vi "Performance Test.vi"() -> ()   [LabVIEW 2021]
uses:
  CIFChannels/Typedef/Direction.ctl
  CIF_NIChn_Fifo_Power_DVR.lvclass
  D:/dev/CIF-LVCore/src/Channels/CIFChannels/CIFChannels.lvclass
  D:/dev/CIF-LVCore/src/Channels/CIF_NIChn/NIChn/CIF_NIChn.lvclass
  ChannelCommon/typedef/FIFO Config.ctl
  <vilib>/Platform/TimedLoop/XDataNode/timing_clust.ctl
  <vilib>/Platform/TimedLoop/XDataNode/nitl_modes.ctl
  <vilib>/Platform/TimedLoop/XDataNode/wakeup.ctl
  ChannelCommon/typedef/TimeStamps.ctl
  ChannelCommon/typedef/Datatype Power Waveform.ctl
  CIF_NIChn_Fifo_Power_DVR.lvclass/CIF_NIChn_Fifo_Power_DVR.ctl
  ChannelCommon/CIFFIFO/CIFfifo.lvclass/CIFfifo.ctl
  NIChn/CIF_NIChn.lvclass/CIF_NIChn.ctl
  CIFChannels/CIFChannels.lvclass/CIFChannels.ctl
  CIFCore/Common/Utilities/Add Error.vi
  SubVIs/Get DVR From Circular Buffer.vi
  Core/Write Power DVR FIFO Direct Dispatch.vi
  Core/Read Power DVR FIFO Direct Dispatch.vi
  CIFCore/Common/Utilities/Append Error Location.vi
  ChannelCommon/Utilities/Get Waveform DVRs.vi
  <vilib>/CIFChannels/Top Level/Write Variable Length U8 Array.vi
  NIChn/Accessors/Read CIF Channel.vi
  NIChn/Accessors/Write CIF Channel.vi
  SubVIs/Flatten.vi
  ChannelCommon/CIFFIFO/Accessors/Read Length.vi
  NIChn/SubVIs/Check Disconnect.vi
  <vilib>/CIFChannels/Top Level/Read Variable Length U8 Array.vi
  SubVIs/Unflatten.vi
  CIFChannels/Accessors/Read Channel State.vi
  CIFChannels/Accessors/Read Direction.vi
  <vilib>/CIFChannels/SubVIs/Get dll Path.vi
  ChannelCommon/CIFFIFO/Utilities/Update Header.vi
  ChannelCommon/CIFFIFO/Flatten/DVR Flatten.vi
  ChannelCommon/CIFFIFO/Accessors/Write T0.vi
  ChannelCommon/CIFFIFO/Accessors/Write T_Out.vi
  ChannelCommon/CIFFIFO/Accessors/Write ClockID.vi
  CIFChannels/Accessors/Write Channel State.vi
  CIFChannels/Accessors/Read Disconnect Behavior.vi
  <vilib>/CIFChannels/Top Level/Read Variable Length U8 Array.vi/81056090-23cf-424a-a716-29db01c8ef1b.vi
  <vilib>/CIFChannels/Top Level/Read Variable Length U8 Array.vi/6610cd62-0a6d-4591-8fd4-6453482a4bc1.vi
  <vilib>/CIFChannels/Top Level/Read Variable Length U8 Array.vi/93d598b0-524b-4f76-9570-a74a86ef2c6f.vi
  ChannelCommon/CIFFIFO/Accessors/Write Timeout.vi
  ChannelCommon/CIFFIFO/Flatten/DVR Unflatten.vi
  ChannelCommon/CIFFIFO/Accessors/Read Header.vi
  ChannelCommon/CIFFIFO/Accessors/Write Header.vi
  ChannelCommon/Utilities/Flatten Header.vi
  ChannelCommon/CIFFIFO/Flatten/DVR Flatten.vi/6fdbece9-bad6-4a8e-9bf7-fe1528478dd6.vi
  ChannelCommon/CIFFIFO/Accessors/Write Payload Length.vi
  <vilib>/CIFChannels/Top Level/Read Variable Length U8 Array.vi/81056090-23cf-424a-a716-29db01c8ef1b.vi/4bc1c15b-36ab-481f-b8dd-c64075ce723a.vi
  <vilib>/CIFChannels/Top Level/Read Variable Length U8 Array.vi/81056090-23cf-424a-a716-29db01c8ef1b.vi/d83cb72b-7713-41fc-a3d1-682de79cf574.vi
  <vilib>/CIFChannels/Top Level/Read Variable Length U8 Array.vi/6610cd62-0a6d-4591-8fd4-6453482a4bc1.vi/c28b0ead-42ad-4072-80a2-aca7f2bd7ce3.vi
  <vilib>/CIFChannels/Top Level/Read Variable Length U8 Array.vi/93d598b0-524b-4f76-9570-a74a86ef2c6f.vi/4bc1c15b-36ab-481f-b8dd-c64075ce723a.vi
  <vilib>/CIFChannels/Top Level/Read Variable Length U8 Array.vi/93d598b0-524b-4f76-9570-a74a86ef2c6f.vi/d83cb72b-7713-41fc-a3d1-682de79cf574.vi
  ChannelCommon/Utilities/Unflatten Header.vi
  ChannelCommon/CIFFIFO/Flatten/DVR Flatten.vi/6fdbece9-bad6-4a8e-9bf7-fe1528478dd6.vi/c28b0ead-42ad-4072-80a2-aca7f2bd7ce3.vi
  NIChn/CIF_NIChn.lvclass
  ChannelCommon/Utilities/Update Time.vi
  <vilib>/Platform/TimedLoop/XDataNode/XDataNode.xnode
  <vilib>/Platform/TimedLoop/XDataNode/XDNodeRunTimeDep.lvlib
  CIFChannels/CIFChannels.lvclass
  ChannelCommon/ChannelCommon.lvlib
panel:
  out "avg TO":dbl
  out "max TO":dbl
  out "timed out? 3":bool
  out "timed out?":bool
  out "avg channel":dbl
  out "max channel":dbl
  out "pass":bool
  out "error out":errorcluster
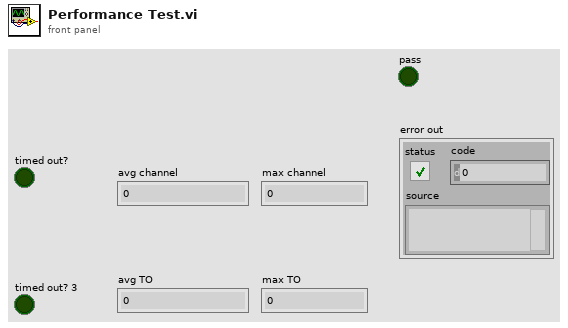
[diagram p1: front panel]
types:
  T1 = typedef "ChannelCommon.lvlib/FIFO Config.ctl" = cluster{"Depth":u64, "Flags":u64, "ClockID":u8}
  T2 = typedef "CIFChannels.lvclass/Direction.ctl" = enum16{"Publisher", "Subscriber"}
  T3 = typedef "ChannelCommon.lvlib/Datatype Power Waveform.ctl" = cluster{"Voltage":dbl[], "Current":dbl[], "dT":dbl, "Timestamp":u64, "Read Lock":bool}
  T4 = typedef "ChannelCommon.lvlib/TimeStamps.ctl" = cluster{"ClockID":u8, "T0":u64, "T_Out":u64}
  T5 = typedef "XDNodeRunTimeDep.lvlib/timing_clust.ctl" = cluster{"Expected End [f-1]":u64, "Actual End [f-1]":u64, "Finished Late? [f-1]":bool, "Expected End [i-1]":u64, "Actual End [i-1]":u64, "Finished Late? [i-1]":bool, "Expected Start [i]":u64, "Actual Start [i]":u64, "Expected Start [f]":u64, "Actual Start [f]":u64, "Source Name":string, "Structure Name":string, "Period":i64, "Deadline":i64, "Offset":i64, "Start":i64, "Priority":i32, "Timeout":i32, "Mode":T6, "Wakeup Reason":T7, "Error":errorcluster, "Source Type":string, "Secondary Source Type":string, "Global End Time":u64, "Global Start Time":u64, "Frame Duration":u64, "Iteration Duration":u64, "Assigned CPU":i32, "I/O Scan Engine Mode":u32}
  T6 = typedef "XDNodeRunTimeDep.lvlib/nitl_modes.ctl" = enum32{"No Change", "Process missed periods, maintain original phase", "Discard missed periods, maintain original phase", "Process missed periods, ignore original phase", "Discard missed periods, ignore original phase"}
  T7 = typedef "XDNodeRunTimeDep.lvlib/wakeup.ctl" = enum32{"Normal", "Aborted", "Asynchronous wakeup", "Timing source error", "Timed loop error", "Timeout"}
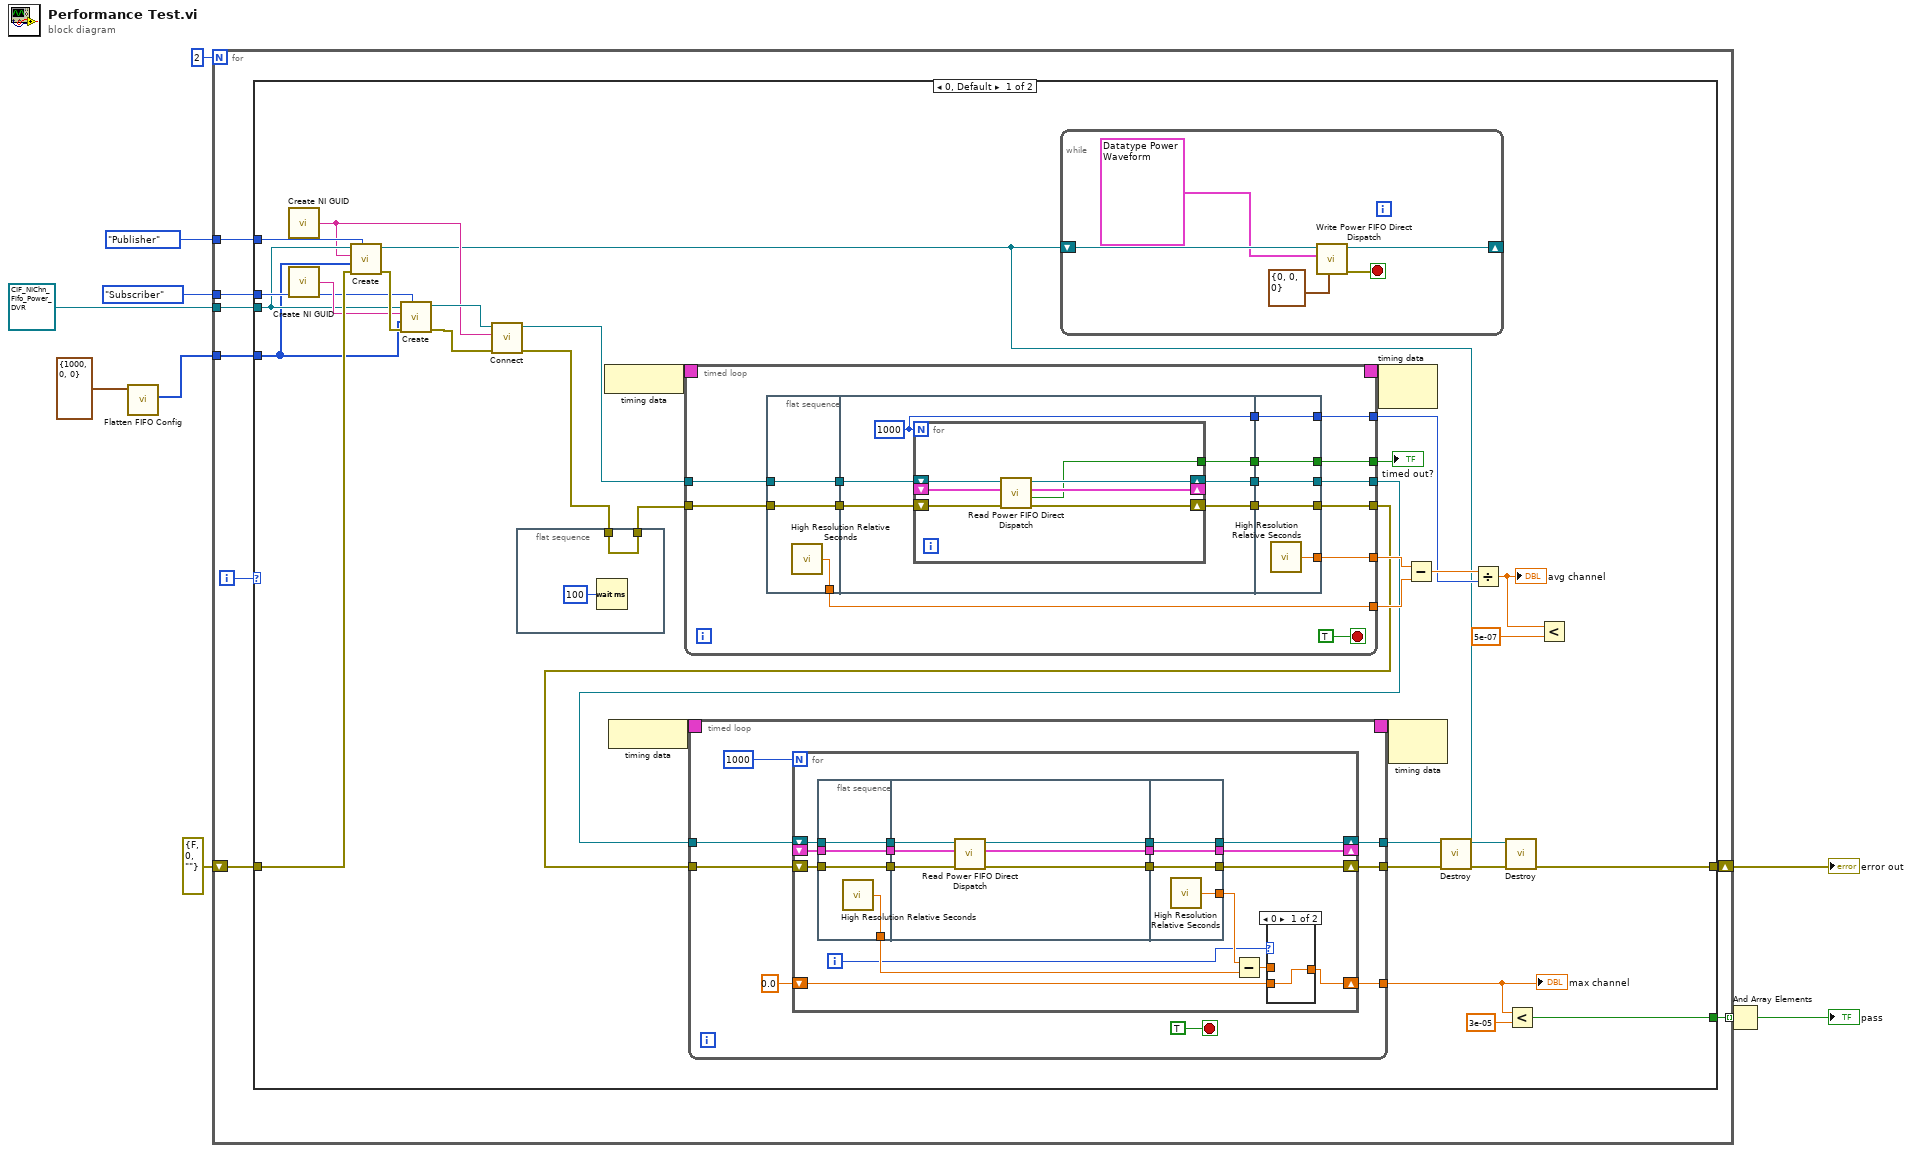
[diagram p0: block diagram]
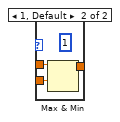
[diagram p2: hidden frame]
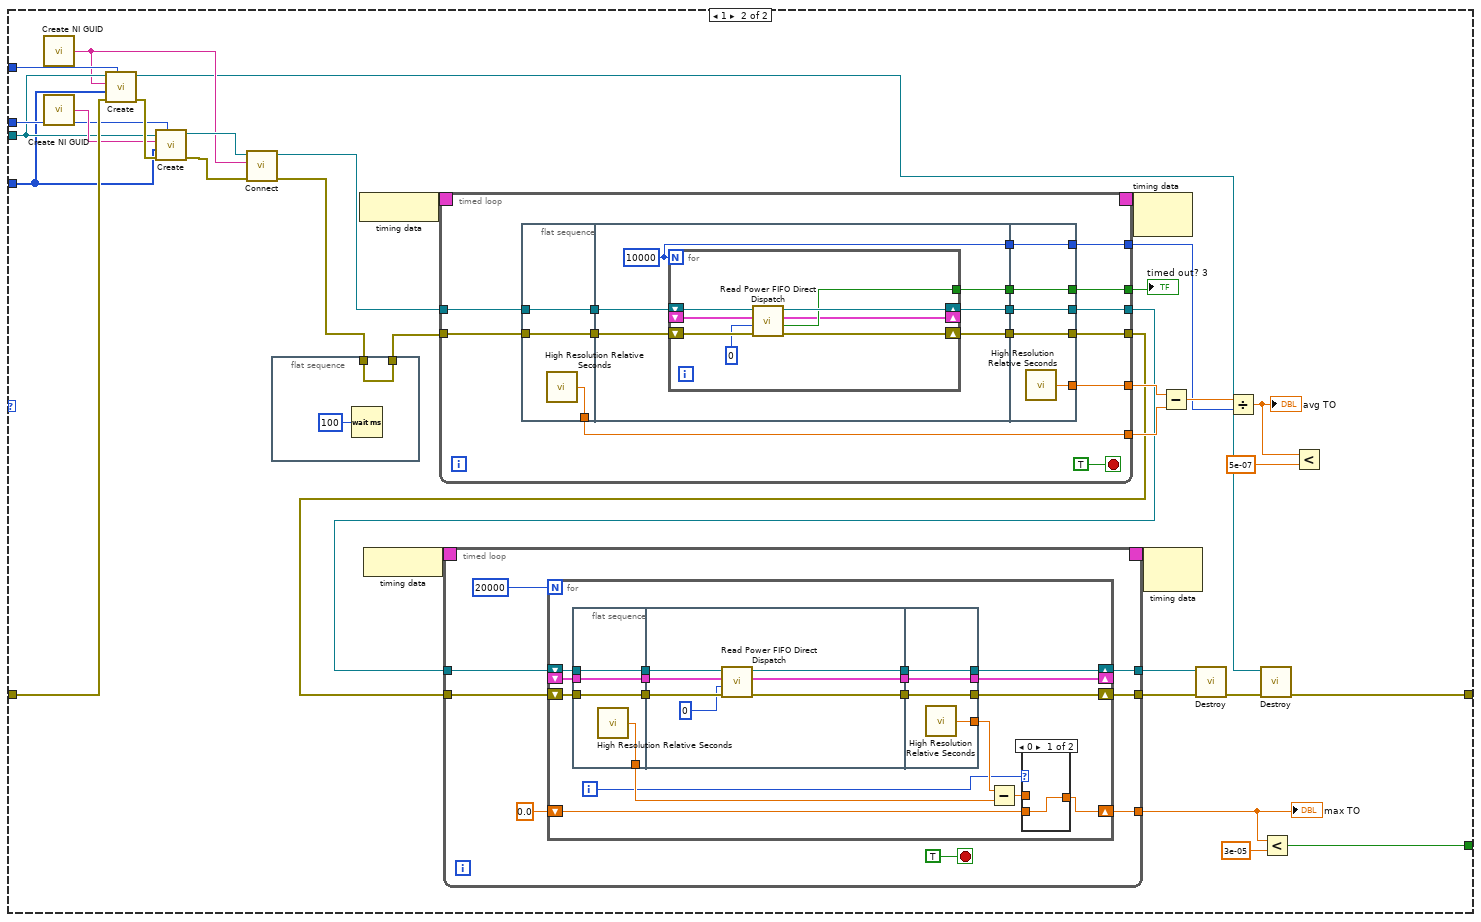
[diagram p3: hidden frame]
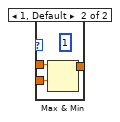
[diagram p4: hidden frame]
diagram:
  n1 = call "Flatten FIFO Config.vi"("FIFO Config in"=T1 {"Depth"=1000, "Flags"=0, "ClockID"=0}) -> ("Flattened Data out"=w2:u8[])  [unwired: 8 in, 2 out]
  n2 = for {
    N: 2 -> [_]
    tunnel: [w18] -> w8 mode=indexing
    shift-right: [w17] -> w10
    shift-left: errorcluster {"status"=FALSE, "code"=0, "source"=""} ("error out") -> [w15]
    tunnel: Direction."Publisher" ("Direction") -> [w14]
    tunnel: Direction."Subscriber" ("Direction") -> [w13]
    tunnel: refnum<class "CIF_NIChn_Fifo_Power_DVR.lvclass"> refnum ("CIF_NIChn_Fifo_Power.lvclass") -> [w12]
    tunnel: w2 -> [w11]
    i -> [w16]
    n3 = case shown="0, Default" w16 {
      tunnel: [w38 w167] -> w18
      tunnel: [w22 w151] -> w17
      tunnel: w15 -> [w36 w165]
      tunnel: w14 -> [w34 w163]
      tunnel: w13 -> [w33 w162]
      tunnel: w12 -> [w32 w161]
      tunnel: w11 -> [w28 w157]
      frame 0, Default {
        n4 = call <vilib>:"Create NI GUID.vi"() -> ("NI GUID"=w30:string)
        n5 = call <vilib>:"Create NI GUID.vi"() -> ("NI GUID"=w35:string)
        n6 = call-dynamic "Create.vi"("Direction"=w34, "error in (no error)"=w36, "Custom Config Data"=w28, "Name"=w30, "CIFTag in"=w32) -> ("error out"=w37:errorcluster, "CIFTag out"=w23:refnum<class "CIF_NIChn_Fifo_Power_DVR.lvclass">)  [unwired: 5 in]
        n7 = call-dynamic "Create.vi"("Direction"=w33, "error in (no error)"=w37, "Custom Config Data"=w28, "Name"=w35, "CIFTag in"=w32) -> ("error out"=w29:errorcluster, "CIFTag out"=w31:refnum<class "CIF_NIChn_Fifo_Power_DVR.lvclass">)  [unwired: 5 in]
        n8 = call-dynamic "Connect.vi"("error in (no error)"=w29, "Connection Name"=w30, "CIFTag in"=w31) -> ("error out"=w21:errorcluster, "CIFTag out"=w27:refnum<class "CIF_NIChn_Fifo_Power_DVR.lvclass">)  [unwired: 7 in]
        n9 = flat-sequence {
          tunnel: w21 -> [w54]
          tunnel: [w54] -> w20
          frame #0 {
            n10 = Wait (ms)(milliseconds to wait=u32 100) -> ()  [unwired: 1 out]
          }
        }
        n11 = node-c288() -> (w52:T5)
        n12 = node-c288() -> (w50:T5)
        n13 = timed-loop {
          timing: w52 -> [_]
          timing-out: [_] -> w51
          tunnel: w27 -> [w122]
          tunnel: w20 -> [w121]
          tunnel: [w117] -> w44
          tunnel: [w115] -> w43
          tunnel: [w113] -> w48
          tunnel: [w112] -> w47
          tunnel: [w111] -> w45
          tunnel: [w109] -> w19
          stop <- TRUE stop-if-true
          n14 = flat-sequence {
            tunnel: w121 -> [w124]
            tunnel: w122 -> [w125]
            tunnel: [w125] -> w119
            tunnel: [w124] -> w118
            tunnel: [w123] -> w112
            tunnel: w119 -> [w131]
            tunnel: w118 -> [w130]
            tunnel: [w129] -> w116
            tunnel: [w128] -> w114
            tunnel: [w127] -> w110
            tunnel: [w126] -> w108
            tunnel: [w143] -> w117
            tunnel: w116 -> [w143]
            tunnel: [w142] -> w115
            tunnel: w114 -> [w142]
            tunnel: [w141] -> w113
            tunnel: [w140] -> w111
            tunnel: w110 -> [w140]
            tunnel: [w139] -> w109
            tunnel: w108 -> [w139]
            frame #0 {
              n15 = call <vilib>:"High Resolution Relative Seconds.vi"() -> ("relative seconds"=w123:dbl)
            }
            frame #1 {
              w127 = 1000
              n16 = for {
                N: w127 -> [_]
                shift-right: [w133] -> w129
                shift-left: w131 -> [w138]
                shift-right: [w136] -> w128
                shift-left: w130 -> [w137]
                shift-right: [w135] -> _
                shift-left: _ -> [w134]
                tunnel: [w132] -> w126
                n17 = call "Read Power FIFO Direct Dispatch.vi"("error in (no error)"=w137, "Power Waveform In"=w134, "CIFTag in"=w138) -> ("error out"=w136:errorcluster, "timed out?"=w132:bool, "Power Waveform Out"=w135:T3, "CIFTag out"=w133:refnum<class "CIF_NIChn_Fifo_Power_DVR.lvclass">)  [unwired: 4 in, 1 out]
              }
            }
            frame #2 {
              n18 = call <vilib>:"High Resolution Relative Seconds.vi"() -> ("relative seconds"=w141:dbl)
            }
          }
        }
        "timed out?" <- w19
        n19 = timed-loop {
          timing: w50 -> [_]
          timing-out: [_] -> w49
          tunnel: w44 -> [w67]
          tunnel: w43 -> [w66]
          tunnel: [w64] -> w26
          tunnel: [w63] -> w25
          tunnel: [w60] -> w40
          stop <- TRUE stop-if-true
          n20 = for {
            N: 1000 -> [_]
            shift-right: [w79] -> w64
            shift-left: w67 -> [w81]
            shift-right: [w78] -> w63
            shift-left: w66 -> [w80]
            shift-right: [w72] -> w60
            shift-left: 0.0 -> [w73]
            shift-right: [w71] -> _
            shift-left: _ -> [w77]
            i -> [w69]
            n21 = flat-sequence {
              tunnel: w80 -> [w92]
              tunnel: w81 -> [w93]
              tunnel: [w93] -> w85
              tunnel: [w92] -> w84
              tunnel: [w91] -> w75
              tunnel: w77 -> [w90]
              tunnel: [w90] -> w83
              tunnel: w85 -> [w99]
              tunnel: w84 -> [w98]
              tunnel: [w95] -> w82
              tunnel: w83 -> [w94]
              tunnel: [w96] -> w70
              tunnel: [w97] -> w68
              tunnel: [w103] -> w79
              tunnel: w82 -> [w103]
              tunnel: [w102] -> w78
              tunnel: [w101] -> w76
              tunnel: [w100] -> w71
              tunnel: w70 -> [w100]
              tunnel: w68 -> [w102]
              frame #0 {
                n22 = call <vilib>:"High Resolution Relative Seconds.vi"() -> ("relative seconds"=w91:dbl)
              }
              frame #1 {
                n23 = call "Read Power FIFO Direct Dispatch.vi"("error in (no error)"=w98, "Power Waveform In"=w94, "CIFTag in"=w99) -> ("error out"=w97:errorcluster, "Power Waveform Out"=w96:T3, "CIFTag out"=w95:refnum<class "CIF_NIChn_Fifo_Power_DVR.lvclass">)  [unwired: 4 in, 2 out]
              }
              frame #2 {
                n24 = call <vilib>:"High Resolution Relative Seconds.vi"() -> ("relative seconds"=w101:dbl)
              }
            }
            n25 = Subtract(x=w76, y=w75) -> (x-y=w74:dbl)
            n26 = case shown="0" w69 {
              tunnel: w74 -> [_ w89]
              tunnel: w73 -> [w86 w88]
              tunnel: [w86 w87] -> w72
              frame 0 {
              }
              frame 1, Default {
                (unwired) u32 1 ("milliseconds to wait")
                n27 = Max & Min(x=w89, y=w88) -> (max(x,y)=w87:dbl)  [unwired: 1 out]
              }
            }
          }
        }
        "max channel" <- w40
        n28 = while {
          shift-right: [w55] -> _
          shift-left: w23 -> [w59]
          stop <- w57 stop-if-true
          n29 = call "Write Power FIFO Direct Dispatch.vi"("FIFO Timestamps"=T4 {"ClockID"=0, "T0"=0, "T_Out"=0}, "Power Waveform In"=T3 {"Voltage"=array[200001 elements], "Current"=array[200001 elements], "dT"=1.0, "Timestamp"=1, "Read Lock"=FALSE}, "CIFTag in"=w59) -> ("error out"=w57:errorcluster, "CIFTag out"=w55:refnum<class "CIF_NIChn_Fifo_Power_DVR.lvclass">)  [unwired: 5 in, 2 out]
        }
        n30 = node-c288(w51) -> ()  [unwired: 1 out]
        n31 = node-c288(w49) -> ()  [unwired: 1 out]
        n32 = Subtract(x=w48, y=w47) -> (x-y=w46:dbl)
        n33 = call-dynamic "Destroy.vi"("error in (no error)"=w25, "CIF_NIChn_Fifo_Power_DVR in"=w26) -> ("error out"=w24:errorcluster)  [unwired: 8 in, 1 out]
        n34 = Divide(x=w46, y=w45) -> (x/y=w42:dbl)
        "avg channel" <- w42
        n35 = call-dynamic "Destroy.vi"("error in (no error)"=w24, "CIF_NIChn_Fifo_Power_DVR in"=w23) -> ("error out"=w22:errorcluster)  [unwired: 8 in, 1 out]
        n36 = Less?(x=w40, y=3e-05) -> (x < y?=w38:bool)
        n37 = Less?(x=w42, y=5e-07) -> ()  [unwired: 1 out]
      }
      frame 1 {
        n38 = call <vilib>:"Create NI GUID.vi"() -> ("NI GUID"=w159:string)
        n39 = call <vilib>:"Create NI GUID.vi"() -> ("NI GUID"=w164:string)
        n40 = call-dynamic "Create.vi"("Direction"=w163, "error in (no error)"=w165, "Custom Config Data"=w157, "Name"=w159, "CIFTag in"=w161) -> ("error out"=w166:errorcluster, "CIFTag out"=w152:refnum<class "CIF_NIChn_Fifo_Power_DVR.lvclass">)  [unwired: 5 in]
        n41 = call-dynamic "Create.vi"("Direction"=w162, "error in (no error)"=w166, "Custom Config Data"=w157, "Name"=w164, "CIFTag in"=w161) -> ("error out"=w158:errorcluster, "CIFTag out"=w160:refnum<class "CIF_NIChn_Fifo_Power_DVR.lvclass">)  [unwired: 5 in]
        n42 = call-dynamic "Connect.vi"("error in (no error)"=w158, "Connection Name"=w159, "CIFTag in"=w160) -> ("error out"=w150:errorcluster, "CIFTag out"=w156:refnum<class "CIF_NIChn_Fifo_Power_DVR.lvclass">)  [unwired: 7 in]
        n43 = flat-sequence {
          tunnel: w150 -> [w183]
          tunnel: [w183] -> w149
          frame #0 {
            n44 = Wait (ms)(milliseconds to wait=u32 100) -> ()  [unwired: 1 out]
          }
        }
        n45 = node-c288() -> (w181:T5)
        n46 = node-c288() -> (w179:T5)
        n47 = timed-loop {
          timing: w181 -> [_]
          timing-out: [_] -> w180
          tunnel: w156 -> [w247]
          tunnel: w149 -> [w246]
          tunnel: [w242] -> w173
          tunnel: [w240] -> w172
          tunnel: [w238] -> w177
          tunnel: [w237] -> w176
          tunnel: [w236] -> w174
          tunnel: [w234] -> w148
          stop <- TRUE stop-if-true
          n48 = flat-sequence {
            tunnel: w246 -> [w249]
            tunnel: w247 -> [w250]
            tunnel: [w250] -> w244
            tunnel: [w249] -> w243
            tunnel: [w248] -> w237
            tunnel: w244 -> [w256]
            tunnel: w243 -> [w255]
            tunnel: [w254] -> w241
            tunnel: [w253] -> w239
            tunnel: [w252] -> w235
            tunnel: [w251] -> w233
            tunnel: [w269] -> w242
            tunnel: w241 -> [w269]
            tunnel: [w268] -> w240
            tunnel: w239 -> [w268]
            tunnel: [w267] -> w238
            tunnel: [w266] -> w236
            tunnel: w235 -> [w266]
            tunnel: [w265] -> w234
            tunnel: w233 -> [w265]
            frame #0 {
              n49 = call <vilib>:"High Resolution Relative Seconds.vi"() -> ("relative seconds"=w248:dbl)
            }
            frame #1 {
              w252 = 10000
              n50 = for {
                N: w252 -> [_]
                shift-right: [w261] -> w254
                shift-left: w256 -> [w264]
                shift-right: [w262] -> w253
                shift-left: w255 -> [w263]
                shift-right: [w259] -> _
                shift-left: _ -> [w258]
                tunnel: [w260] -> w251
                n51 = call "Read Power FIFO Direct Dispatch.vi"("error in (no error)"=w263, "Timeout (ms)"=0, "Power Waveform In"=w258, "CIFTag in"=w264) -> ("error out"=w262:errorcluster, "timed out?"=w260:bool, "Power Waveform Out"=w259:T3, "CIFTag out"=w261:refnum<class "CIF_NIChn_Fifo_Power_DVR.lvclass">)  [unwired: 3 in, 1 out]
              }
            }
            frame #2 {
              n52 = call <vilib>:"High Resolution Relative Seconds.vi"() -> ("relative seconds"=w267:dbl)
            }
          }
        }
        "timed out? 3" <- w148
        n53 = timed-loop {
          timing: w179 -> [_]
          timing-out: [_] -> w178
          tunnel: w173 -> [w191]
          tunnel: w172 -> [w190]
          tunnel: [w188] -> w155
          tunnel: [w187] -> w154
          tunnel: [w184] -> w169
          stop <- TRUE stop-if-true
          n54 = for {
            N: 20000 -> [_]
            shift-right: [w203] -> w188
            shift-left: w191 -> [w205]
            shift-right: [w202] -> w187
            shift-left: w190 -> [w204]
            shift-right: [w196] -> w184
            shift-left: 0.0 -> [w197]
            shift-right: [w195] -> _
            shift-left: _ -> [w201]
            i -> [w193]
            n55 = flat-sequence {
              tunnel: w204 -> [w216]
              tunnel: w205 -> [w217]
              tunnel: [w217] -> w209
              tunnel: [w216] -> w208
              tunnel: [w215] -> w199
              tunnel: w201 -> [w214]
              tunnel: [w214] -> w207
              tunnel: w209 -> [w224]
              tunnel: w208 -> [w220]
              tunnel: [w223] -> w206
              tunnel: w207 -> [w221]
              tunnel: [w222] -> w194
              tunnel: [w219] -> w192
              tunnel: [w228] -> w203
              tunnel: w206 -> [w228]
              tunnel: [w227] -> w202
              tunnel: [w226] -> w200
              tunnel: [w225] -> w195
              tunnel: w194 -> [w225]
              tunnel: w192 -> [w227]
              frame #0 {
                n56 = call <vilib>:"High Resolution Relative Seconds.vi"() -> ("relative seconds"=w215:dbl)
              }
              frame #1 {
                n57 = call "Read Power FIFO Direct Dispatch.vi"("error in (no error)"=w220, "Timeout (ms)"=0, "Power Waveform In"=w221, "CIFTag in"=w224) -> ("error out"=w219:errorcluster, "Power Waveform Out"=w222:T3, "CIFTag out"=w223:refnum<class "CIF_NIChn_Fifo_Power_DVR.lvclass">)  [unwired: 3 in, 2 out]
              }
              frame #2 {
                n58 = call <vilib>:"High Resolution Relative Seconds.vi"() -> ("relative seconds"=w226:dbl)
              }
            }
            n59 = Subtract(x=w200, y=w199) -> (x-y=w198:dbl)
            n60 = case shown="0" w193 {
              tunnel: w198 -> [_ w213]
              tunnel: w197 -> [w210 w212]
              tunnel: [w210 w211] -> w196
              frame 0 {
              }
              frame 1, Default {
                (unwired) u32 1 ("milliseconds to wait")
                n61 = Max & Min(x=w213, y=w212) -> (max(x,y)=w211:dbl)  [unwired: 1 out]
              }
            }
          }
        }
        "max TO" <- w169
        n62 = node-c288(w180) -> ()  [unwired: 1 out]
        n63 = node-c288(w178) -> ()  [unwired: 1 out]
        n64 = Subtract(x=w177, y=w176) -> (x-y=w175:dbl)
        n65 = call-dynamic "Destroy.vi"("error in (no error)"=w154, "CIF_NIChn_Fifo_Power_DVR in"=w155) -> ("error out"=w153:errorcluster)  [unwired: 8 in, 1 out]
        n66 = Divide(x=w175, y=w174) -> (x/y=w171:dbl)
        "avg TO" <- w171
        n67 = call-dynamic "Destroy.vi"("error in (no error)"=w153, "CIF_NIChn_Fifo_Power_DVR in"=w152) -> ("error out"=w151:errorcluster)  [unwired: 8 in, 1 out]
        n68 = Less?(x=w169, y=3e-05) -> (x < y?=w167:bool)
        n69 = Less?(x=w171, y=5e-07) -> ()  [unwired: 1 out]
      }
    }
  }
  "error out" <- w10
  n70 = And Array Elements(Boolean array=w8) -> (logical AND=→"pass":bool)
